vi "CleanUp.vi"(8 "Error In":errorcluster, 11 "Object in":refnum<class "PXIe-5172.lvclass">) -> (0 "Error Out":errorcluster, 3 "object out":refnum<class "PXIe-5172.lvclass">)   [LabVIEW 2023, in "HAL.lvlib" / "PXIe-5172.lvlib" / "PXIe-5172.lvclass"]
uses:
  PXIe-5172.lvclass
  PXIe-5172.lvclass/PXIe-5172.ctl
  Hardware_class/Hardware.lvclass
  <resource>/Framework/Providers/Open_GDS/ClassProviders/Provider_LvNativeClass/Templates/NativeSubTemplate_4x4x4/NativeSubTemplate_4x4x4.lvclass
  C:/Program Files/National Instruments/LabVIEW 2023/resource/Framework/Providers/Open_GDS/ClassProviders/Provider_LvNativeClass/Templates/NativeBaseTemplate_4x4x4/NativeBaseTemplate_4x4x4.lvclass
  C:/Program Files/National Instruments/LabVIEW 2023/resource/Framework/Providers/Open_GDS/ClassProviders/Provider_LvNativeClass/Templates/NativeSubTemplate_4x4x4/NativeSubTemplate_4x4x4.lvclass
  D:/git/HAL/Hardware_class/Hardware.lvclass
  D:/git/HAL/PXIe-5172_class/PXIe-5172.lvclass
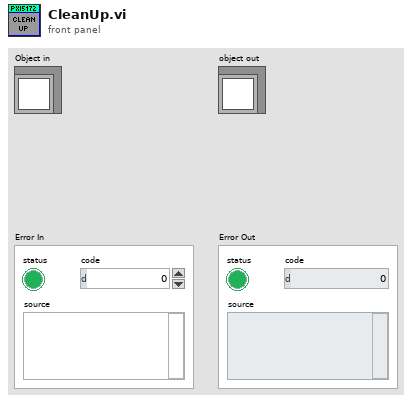
[diagram p1: front panel]
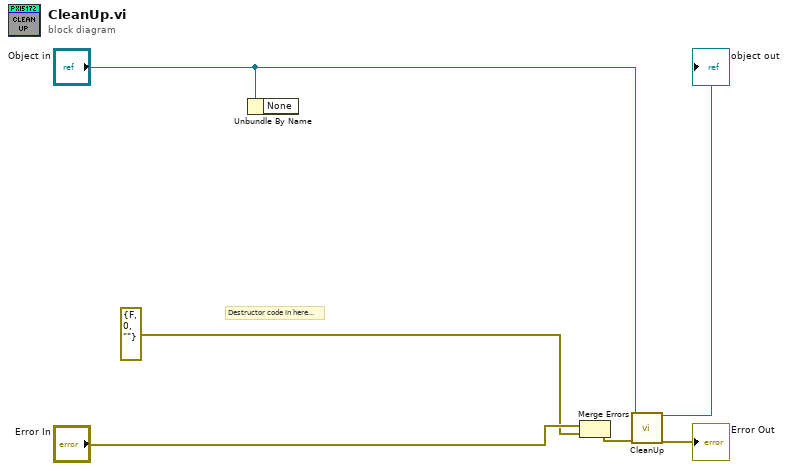
[diagram p0: block diagram]
diagram:
  # "Destructor code in here..."
  n1 = Unbundle By Name("Object in") -> ()  [unwired: 1 out]
  n2 = Merge Errors("Error In", errorcluster {"status"=FALSE, "code"=0, "source"=""} ("error in (no error)")) -> (w2:errorcluster)
  n3 = call-parent "CleanUp.vi"("Error In"=w2, "object in"="Object in") -> ("Error Out"=→"Error Out":errorcluster, "object out"=→"object out":refnum<class "NativeSubTemplate_4x4x4.lvclass">)  [unwired: 8 in]
